vi "Check Pattern Name with CSV name.vi"(8 "error in (no error)":errorcluster, 10 "Data Array out":T1[](array[typedef]) {"Data" format="%x"; "Start_Addr" format="%x"}, 11 "Path":path) -> (0 "error out":errorcluster)   [LabVIEW 2018, in "Config_Read_BML.lvclass"]
uses:
  Config_Read_BML.lvclass
  Frame_Data.ctl
  OperationMode.ctl
  BurstLength.ctl
  RW_Option.ctl
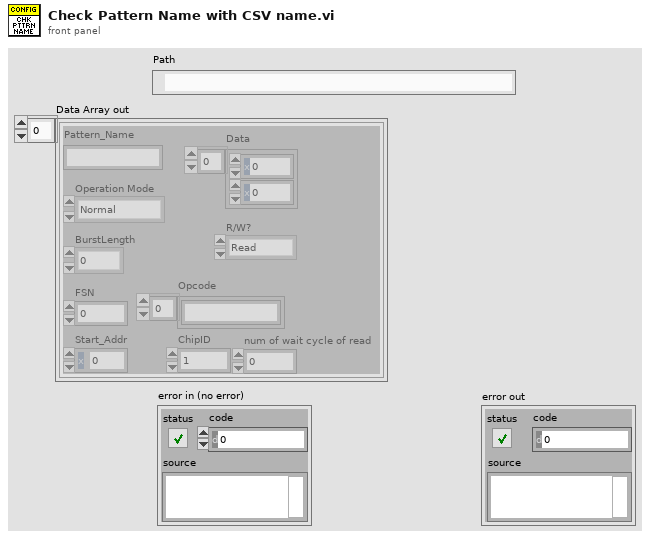
[diagram p1: front panel]
types:
  T1 = typedef "Config_Read_BML.lvclass/Frame_Data.ctl" = cluster{"Pattern_Name":string, "Operation Mode":T2, "BurstLength":T3, "FSN":u8, "Start_Addr":u16, "Data":u8[], "R/W?":T4, "Opcode":string[], "ChipID":u8, "num of wait cycle of read":i8}
  T2 = typedef "Config_Read_BML.lvclass/OperationMode.ctl" = enum8{"Normal", "ImmeEffect", "InitSlaveID", "LoadData"}
  T3 = typedef "Config_Read_BML.lvclass/BurstLength.ctl" = enum8{"0", "2", "3", "4", "5", "8", "16", "32"}
  T4 = typedef "Config_Read_BML.lvclass/RW_Option.ctl" = enum16{"Read", "Write", "R/W"}
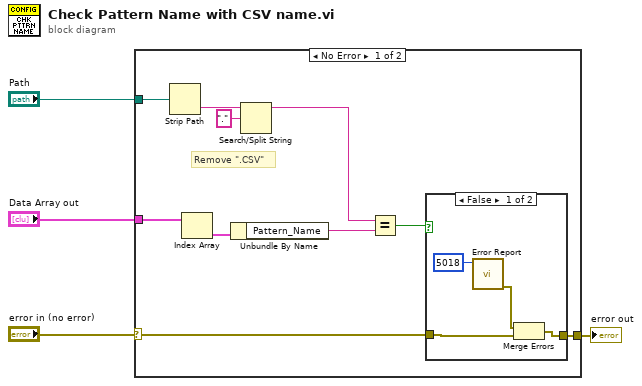
[diagram p0: block diagram]
diagram:
  n1 = case shown="No Error" "error in (no error)" {
    selector: "error in (no error)" -> [w9 w20]
    tunnel: "Data Array out" -> [w13 _]
    tunnel: "Path" -> [w14 _]
    tunnel: [w8 w20] -> w1
    frame No Error {
      # "Remove \".CSV\""
      n2 = Strip Path(path=w14) -> (name=w7:string)  [unwired: 1 out]
      n3 = Index Array(array=w13) -> (element=w12:T1)  [unwired: 1 in]
      n4 = Unbundle By Name(w12) -> ("Pattern_Name"=w11:string)
      n5 = Search/Split String(string=w7, search string/char (-)=".") -> (substring before match=w5:string)  [unwired: 1 in, 2 out]
      n6 = Equal?(x=w5, y=w11) -> (x = y?=w10:bool)
      n7 = case shown="False" w10 {
        tunnel: w9 -> [w16 w19]
        tunnel: [w15 w19] -> w8
        frame False {
          n8 = call "Error Report.vi"("Error Code"=i16 5018) -> ("error out"=w17:errorcluster)  [unwired: 10 in]
          n9 = Merge Errors(w17, w16) -> (w15:errorcluster)
        }
        frame True {
        }
      }
    }
    frame Error {
    }
  }
  "error out" <- w1
